vi "Init.vi"(8 "error in (no error)":errorcluster, 11 "Soda Actors in":refnum<class "Soda Actors.lvclass">) -> (0 "error out":errorcluster, 3 "Soda Actors out":refnum<class "Soda Actors.lvclass">)   [LabVIEW 2020, in "Soda Actors.lvlib" / "Soda Actors.lvclass"]
uses:
  Soda Actors.lvclass
  Soda Actors.lvclass/Soda Actors.ctl
  <vilib>/Utility/config.llb/Read Key (Double).vi
  <vilib>/Utility/config.llb/Read Key (String).vi
  <vilib>/Utility/config.llb/NI_LVConfig.lvlib
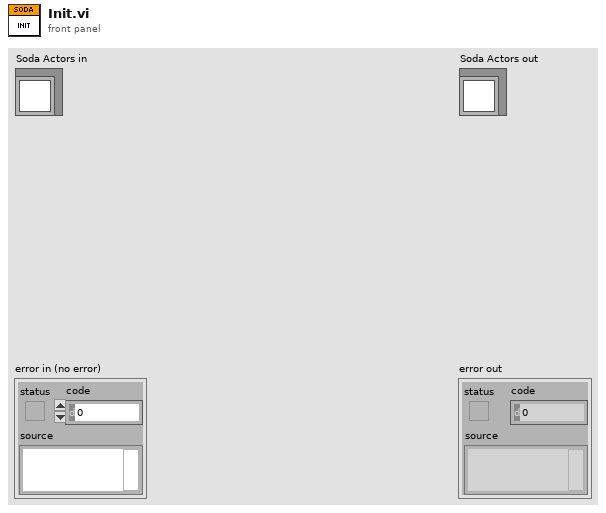
[diagram p1: front panel]
types:
  T1 = typedef "NI_LVConfig.lvlib/Config Data RefNum.ctl" = refnum<k1>
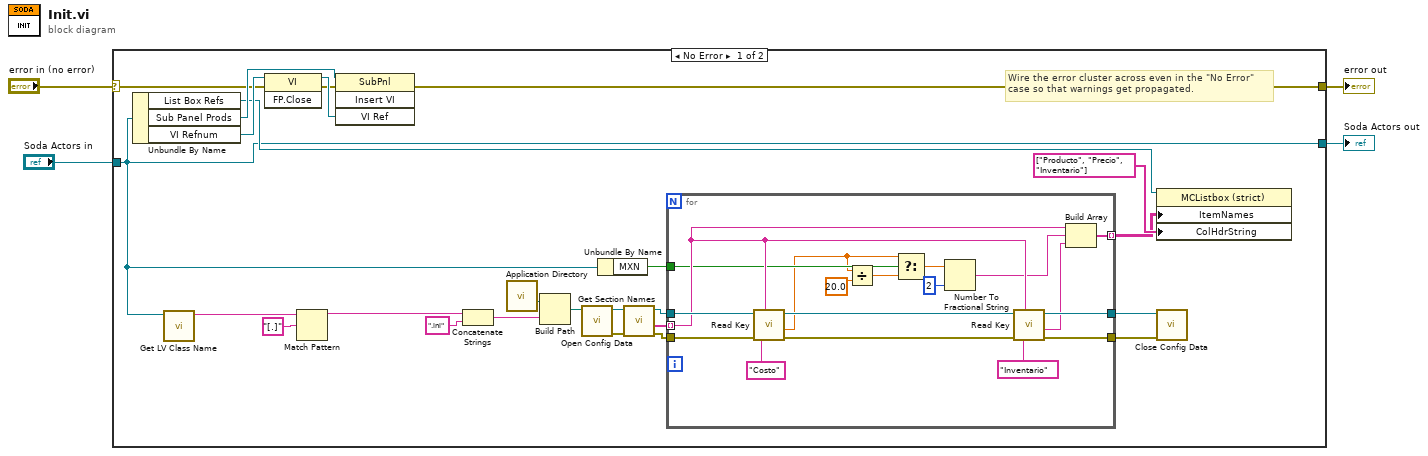
[diagram p0: block diagram]
diagram:
  n1 = case shown="No Error" "error in (no error)" {
    selector: "error in (no error)" -> [w25 w49]
    tunnel: [w24 w49] -> w3
    tunnel: [w12 w48] -> w1
    tunnel: "Soda Actors in" -> [w12 w48]
    frame No Error {
      # "Wire the error cluster across even in the \"No Error\"\ncase so that warnings get propagated."
      n2 = Unbundle By Name(w12) -> ("List Box Refs"=w23:refnum<vi>, "Sub Panel Prods"=w26:refnum<vi>, "VI Refnum"=w27:refnum<vi>)
      n3 = call <vilib>:"Get LV Class Name.vi"("object"=w12) -> ("class name"=w15:string)  [unwired: 9 in, 1 out]
      n4 = invoke class="VI" method="FP.Close"(reference=w27, error in=w25) -> (reference out=w29:refnum<vi>, error out=w28:errorcluster)  [unwired: 1 in, 1 out]
      n5 = Match Pattern(string=w15, regular expression="[.]") -> (before substring=w13:string)  [unwired: 1 in, 3 out]
      n6 = invoke class="SubPnl" method="Insert VI"(reference=w26, error in=w28, "VI Ref"=w29) -> (error out=w24:errorcluster)  [unwired: 1 in, 3 out]
      n7 = Concatenate Strings(w13, ".ini" ("string")) -> (w20:string)
      n8 = call <vilib>:"Application Directory.vi"() -> ("Application Directory"=w22:path)
      n9 = Build Path(base path=w22, name or relative path=w20) -> (appended path=w19:path)
      n10 = call <vilib>:"Open Config Data.vi"("configuration file path"=w19) -> ("error out"=w18:errorcluster, "refnum"=w9:T1)  [unwired: 8 in, 1 out]
      n11 = Unbundle By Name(w12) -> ("MXN"=w11:bool)
      n12 = call <vilib>:"Get Section Names.vi"("error in (no error)"=w18, "refnum"=w9) -> ("error out"=w10:errorcluster, "section names"=w7:string[], "refnum out"=w8:T1)  [unwired: 7 in]
      n13 = for {
        tunnel: w8 -> [w47]
        tunnel: w10 -> [w46]
        tunnel: [w43] -> w17
        tunnel: [w42] -> w16
        tunnel: w11 -> [w34]
        tunnel: w7 -> [w40] mode=indexing
        tunnel: [w38] -> w5 mode=indexing
        n14 = call-poly <vilib>:"Read Key.vi"("section"=w40, "error in (no error)"=w46, "key"="Costo", "refnum"=w47) -> ("error out"=w45:errorcluster, "value"=w30:dbl, "refnum out"=w44:T1)  [unwired: 4 in, 1 out]
        n15 = Divide(x=w30, y=20.0) -> (x/y=w32:dbl)
        n16 = Select(t=w30, s=w34, f=w32) -> (s? t:f=w33:dbl)
        n17 = Number To Fractional String(number=w33, precision (6)=i16 2) -> (F-format string=w36:string)  [unwired: 2 in]
        n18 = call-poly <vilib>:"Read Key.vi"("section"=w40, "error in (no error)"=w45, "key"="Inventario", "refnum"=w44) -> ("error out"=w43:errorcluster, "value"=w39:string, "refnum out"=w42:T1)  [unwired: 4 in, 1 out]
        n19 = Build Array(w40, w36, w39) -> (w38:string[])
      }
      n20 = property class="MCListbox (strict)"(reference=w23, "ItemNames"=w5, "ColHdrString"=string[] ["Producto", "Precio", "Inventario"] ("Column Header Strings[]")) -> ()  [unwired: 1 in, 2 out]
      n21 = call <vilib>:"Close Config Data.vi"("error in (no error)"=w17, "refnum"=w16) -> ()  [unwired: 8 in, 2 out]
    }
    frame Error {
    }
  }
  "error out" <- w3
  "Soda Actors out" <- w1
